vi "ZMC Get Max Pci Cards.vi"(8 "error in (no error)":errorcluster caption="错误输入（无错误）") -> (0 "error out":errorcluster caption="错误输出", 3 "function return":u32)   [LabVIEW 2015, in "zauxdll.lvlib"]
doc: "uint32 __stdcall ZMC_GetMaxPciCards();"
uses:
  zauxdll.lvlib
  zmotion.dll
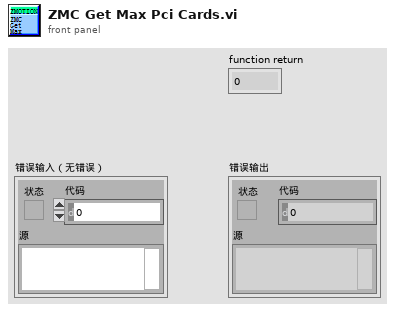
[diagram p1: front panel]
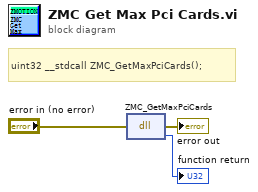
[diagram p0: block diagram]
diagram:
  # "uint32 __stdcall ZMC_GetMaxPciCards();"
  n1 = dll-call lib="C:/Users/VIC/Desktop/GOGORO_SA/system/LLB/zmotion/zaux/zmotion.*" fn="ZMC_GetMaxPciCards"(error in="error in (no error)") -> (error out=→"error out":errorcluster, →"function return":u32)  [unwired: 2 in, 1 out]
